vi "Get ECAT Variable Contents.vi"(8 "error in (no error)":errorcluster, 11 "ECAT Variablenobjekt in":refnum<k21>[](array[refnum])) -> (0 "error out":errorcluster, 2 "All Variables Contents":T1[](array[typedef]), 3 "ECAT Variablenobjekt out":refnum<k21>[](array[refnum]))   [LabVIEW 2019, in "SEECD System Explorer.lvlib"]
uses:
  SEECD System Explorer.lvlib
  Type Defs/IOV Container Contents.ctl
  <resource>/objmgr/ni.var.rc
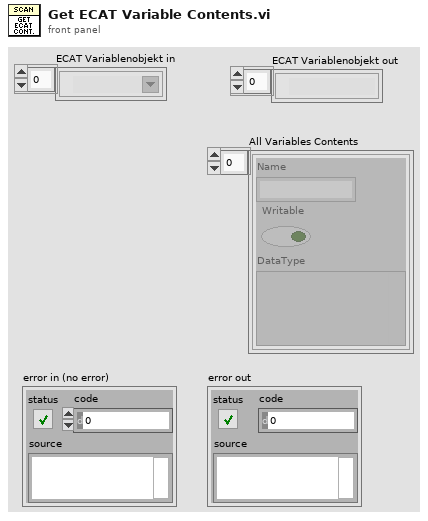
[diagram p1: front panel]
types:
  T1 = typedef "SEECD System Explorer.lvlib/IOV Container Contents.ctl" = cluster{"Name":string, "Writable":bool, "DataType":variant}
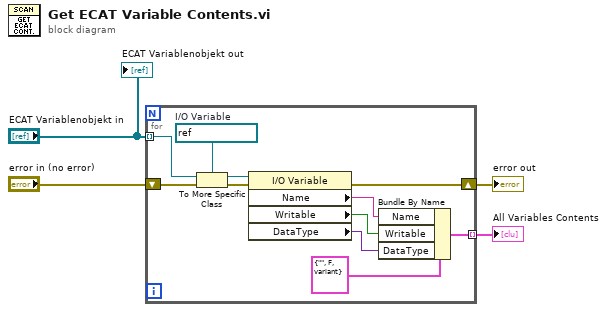
[diagram p0: block diagram]
diagram:
  n1 = for {
    tunnel: "ECAT Variablenobjekt in" -> [w7] mode=indexing
    shift-right: [w15] -> w4
    shift-left: "error in (no error)" -> [w8]
    tunnel: [w10] -> w3 mode=indexing
    w9 = refnum<k21> refnum  # I/O Variable
    n2 = To More Specific Class(target class=w9, reference=w7, error in=w8) -> (specific class reference=w6:refnum<k21>, error out=w5:errorcluster)
    n3 = property class="I/O Variable"(reference=w6, error in=w5) -> (error out=w15:errorcluster, "Name"=w13:string, "Writable"=w12:bool, "DataType"=w11:variant)  [unwired: 1 out]
    n4 = Bundle By Name(cluster=T1 {"Name"="", "Writable"=FALSE, "DataType"=variant} ("IO Variable Container Contents"), "Name"=w13, "Writable"=w12, "DataType"=w11) -> (w10:T1)
  }
  "error out" <- w4
  "All Variables Contents" <- w3
  "ECAT Variablenobjekt out" <- "ECAT Variablenobjekt in"
